vi "next_step.vi"(5 "premove":dbl, 7 "penter":dbl, 8 "keep":dbl[](array[numeric]), 9 "in":dbl[](array[numeric]), 10 "PVal":dbl[](array[numeric]), 11 "B":dbl[](array[numeric])) -> (0 "swap":dbl, 3 "p":dbl)   [LabVIEW 2014]
panel:
  out "kmin":i32
  out "pmin":dbl
  out "termsout":i32[](array[numeric])
  # "INPUT"
  # "P, SWAP"
  # "termsout"
  # "pmin/kmin"
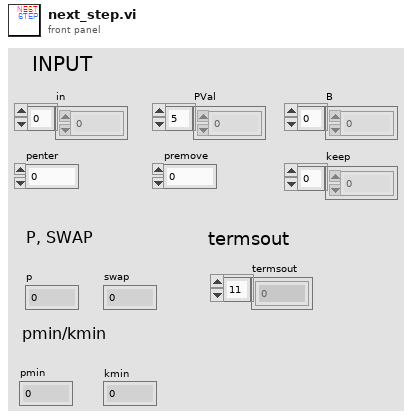
[diagram p1: front panel]
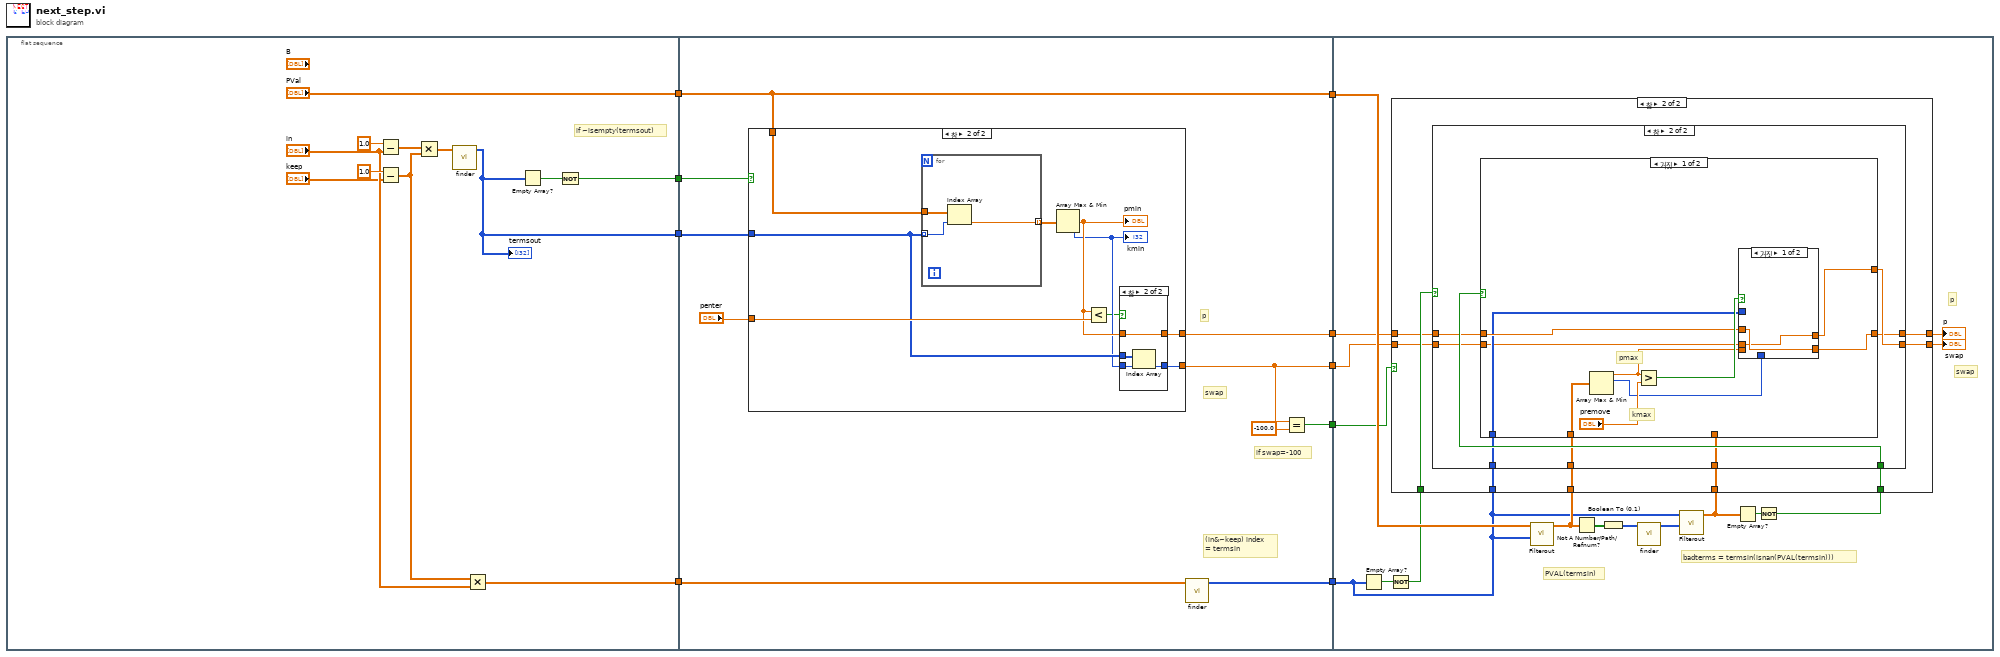
[diagram p0: block diagram]
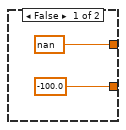
[diagram p2: hidden frame]
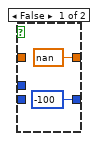
[diagram p3: hidden frame]
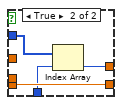
[diagram p6: hidden frame]
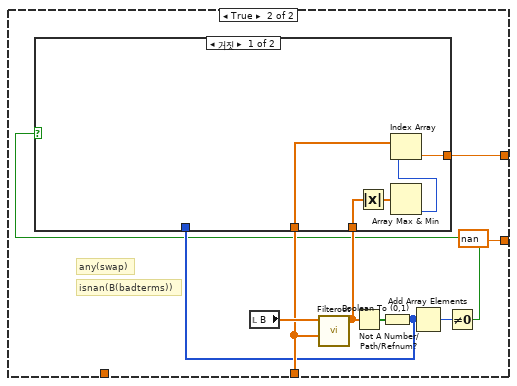
[diagram p7: hidden frame]
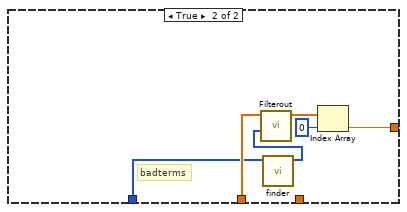
[diagram p8: hidden frame]
diagram:
  n1 = flat-sequence {
    tunnel: ["PVal"] -> w9
    tunnel: [w16] -> w8
    tunnel: [w12] -> w7
    tunnel: [w14] -> w5
    tunnel: w9 -> [w27]
    tunnel: w8 -> [w25]
    tunnel: w7 -> [w31]
    tunnel: [w23] -> w6
    tunnel: w5 -> [w29]
    tunnel: [w28] -> w4
    tunnel: [w27] -> w3
    tunnel: [w26] -> w2
    tunnel: [w24] -> w1
    tunnel: w6 -> [w59]
    tunnel: w4 -> [w56]
    tunnel: w3 -> [w63]
    tunnel: w2 -> [w58]
    tunnel: w1 -> [w52]
    frame #0 {
      # "if ~isempty(termsout)"
      n2 = Subtract(x=1.0, y="in") -> (x-y=w19:dbl[])
      n3 = Subtract(x=1.0, y="keep") -> (x-y=w15:dbl[])
      n4 = Multiply(x=w19, y=w15) -> (x*y=w18:dbl[])
      n5 = call "finder.vi"("Array 3"=w18) -> ("Array out"=w12:i32[])  [unwired: 10 in]
      "termsout" <- w12
      n6 = Multiply(x=w15, y="in") -> (x*y=w14:dbl[])
      n7 = Empty Array?(array=w12) -> (empty?=w13:bool)
      n8 = Not(x=w13) -> (.not. x?=w16:bool)
    }
    frame #1 {
      # "if swap=-100"
      # "(in&~keep) index\n= termsin"
      # "swap"
      # "p"
      n9 = case shown="참" w25 {
        tunnel: w27 -> [_ w36]
        tunnel: w31 -> [_ w41]
        tunnel: "penter" -> [_ w42]
        tunnel: [nan w38] -> w26
        tunnel: [-100.0 w37] -> w23
        frame False {
        }
        frame True {
          n10 = for {
            tunnel: w41 -> [w50] mode=indexing
            tunnel: w36 -> [w51]
            tunnel: [w49] -> w34 mode=indexing
            n11 = Index Array(array=w51, index=w50) -> (element=w49:dbl)
          }
          n12 = Array Max & Min(array=w34) -> (min value=w40:dbl, min index (indices)=w39:i32)  [unwired: 2 out]
          "pmin" <- w40
          "kmin" <- w39
          n13 = Less?(x=w40, y=w42) -> (x < y?=w35:bool)
          n14 = case shown="참" w35 {
            tunnel: w41 -> [_ w47]
            tunnel: w40 -> [_ w48]
            tunnel: [nan w48] -> w38
            tunnel: w39 -> [_ w46]
            tunnel: [-100 w45] -> w37
            frame False {
            }
            frame True {
              n15 = Index Array(array=w47, index=w46) -> (element=w45:i32)
            }
          }
        }
      }
      n16 = call "finder.vi"("Array 3"=w29) -> ("Array out"=w28:i32[])  [unwired: 10 in]
      n17 = Equal?(x=w23, y=-100.0) -> (x = y?=w24:bool)
    }
    frame #2 {
      # "swap"
      # "p"
      # "badterms = termsin(isnan(PVAL(termsin)))"
      # "PVAL(termsin)"
      n18 = Empty Array?(array=w56) -> (empty?=w67:bool)
      n19 = Not(x=w67) -> (.not. x?=w53:bool)
      n20 = call "Filterout.vi"("elements"=w56, "Array"=w63) -> ("output"=w57:dbl[])  [unwired: 9 in]
      n21 = Not A Number/Path/Refnum?(number/path/refnum=w57) -> (NaN/Path/Refnum?=w64:bool[])
      n22 = Boolean To (0,1)(Boolean=w64) -> (0, 1=w65:i16[])
      n23 = call "finder.vi"("Array 3"=w65) -> ("Array out"=w66:i32[])  [unwired: 10 in]
      n24 = call "Filterout.vi"("elements"=w66, "Array"=w56) -> ("output"=w60:dbl[])  [unwired: 9 in]
      n25 = Empty Array?(array=w60) -> (empty?=w62:bool)
      n26 = Not(x=w62) -> (.not. x?=w61:bool)
      n27 = case shown="참" w52 {
        tunnel: w53 -> [_ w78]
        tunnel: w61 -> [_ w77]
        tunnel: w60 -> [_ w76]
        tunnel: w59 -> [w69 w75]
        tunnel: [w69 w74] -> w54
        tunnel: w58 -> [w68 w73]
        tunnel: [w68 w72] -> w55
        tunnel: w57 -> [_ w71]
        tunnel: w56 -> [_ w70]
        frame False {
        }
        frame True {
          n28 = case shown="참" w78 {
            tunnel: w77 -> [_ w88]
            tunnel: w76 -> [_ w87]
            tunnel: [w80 w86] -> w74
            tunnel: w75 -> [w80 w81]
            tunnel: w73 -> [w79 w83]
            tunnel: [w79 w85] -> w72
            tunnel: w71 -> [_ w84]
            tunnel: w70 -> [_ w82]
            frame False {
            }
            frame True {
              n29 = case shown="거짓" w88 {
                tunnel: w87 -> [_ w111]
                tunnel: [w90 w109] -> w86
                tunnel: [w94 nan] -> w85
                tunnel: w84 -> [w98 _]
                tunnel: w83 -> [w93 _]
                tunnel: w82 -> [w92 _]
                tunnel: w81 -> [w89 _]
                frame False {
                  # "kmax"
                  # "pmax"
                  n30 = Array Max & Min(array=w98) -> (max value=w95:dbl, max index (indices)=w91:i32)  [unwired: 2 out]
                  n31 = Greater?(x=w95, y="premove") -> (0:w96:bool)
                  n32 = case shown="거짓" w96 {
                    tunnel: w95 -> [_ w104]
                    tunnel: [w100 w104] -> w94
                    tunnel: w93 -> [w100 _]
                    tunnel: w92 -> [_ w103]
                    tunnel: w91 -> [_ w102]
                    tunnel: [w99 w101] -> w90
                    tunnel: w89 -> [w99 _]
                    frame False {
                    }
                    frame True {
                      n33 = Index Array(array=w103, index=w102) -> (element=w101:i32)
                    }
                  }
                }
                frame True {
                  # "any(swap)"
                  # "isnan(B(badterms))"
                  n34 = local read "B"() -> (w113:dbl[])
                  n35 = call "Filterout.vi"("elements"=w111, "Array"=w113) -> ("output"=w108:dbl[])  [unwired: 9 in]
                  n36 = Not A Number/Path/Refnum?(number/path/refnum=w108) -> (NaN/Path/Refnum?=w112:bool[])
                  n37 = Boolean To (0,1)(Boolean=w112) -> (0, 1=w110:i16[])
                  n38 = Add Array Elements(numeric array=w110) -> (sum=w106:i16)
                  n39 = Not Equal To 0?(x=w106) -> (x != 0?=w105:bool)
                  n40 = case shown="거짓" w105 {
                    tunnel: w111 -> [w116 w124]
                    tunnel: w110 -> [_ w122]
                    tunnel: [w114 w119] -> w109
                    tunnel: w108 -> [w118 _]
                    frame False {
                      n41 = Absolute Value(x=w118) -> (abs(x)=w117:dbl[])
                      n42 = Array Max & Min(array=w117) -> (min index (indices)=w115:i32)  [unwired: 3 out]
                      n43 = Index Array(array=w116, index=w115) -> (element=w114:dbl)
                    }
                    frame True {
                      # "badterms"
                      n44 = call "finder.vi"("Array 3"=w122) -> ("Array out"=w123:i32[])  [unwired: 10 in]
                      n45 = call "Filterout.vi"("elements"=w123, "Array"=w124) -> ("output"=w121:dbl[])  [unwired: 9 in]
                      n46 = Index Array(array=w121, index=0) -> (element=w119:dbl)
                    }
                  }
                }
              }
            }
          }
        }
      }
      "p" <- w55
      "swap" <- w54
    }
  }
